vi "Example Interrupt.vi"() -> ()   [LabVIEW 2013]
uses:
  C:/tf/play/labview/Tinkerforge.dll
panel:
  out "value mask":bool[](array[boolean])
  out "interrupt mask":bool[](array[boolean])
  in  "stop":bool
  in  "uid":string="aE7"
  in  "port":i32=4223
  in  "host":string="localhost"
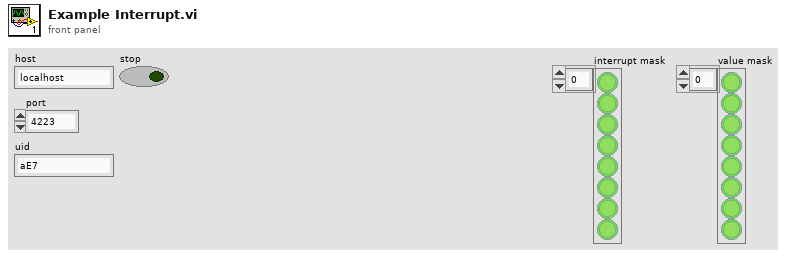
[diagram p1: front panel]
types:
  T1 = cluster{"port":u16, "interruptMask":u8, "valueMask":u8}
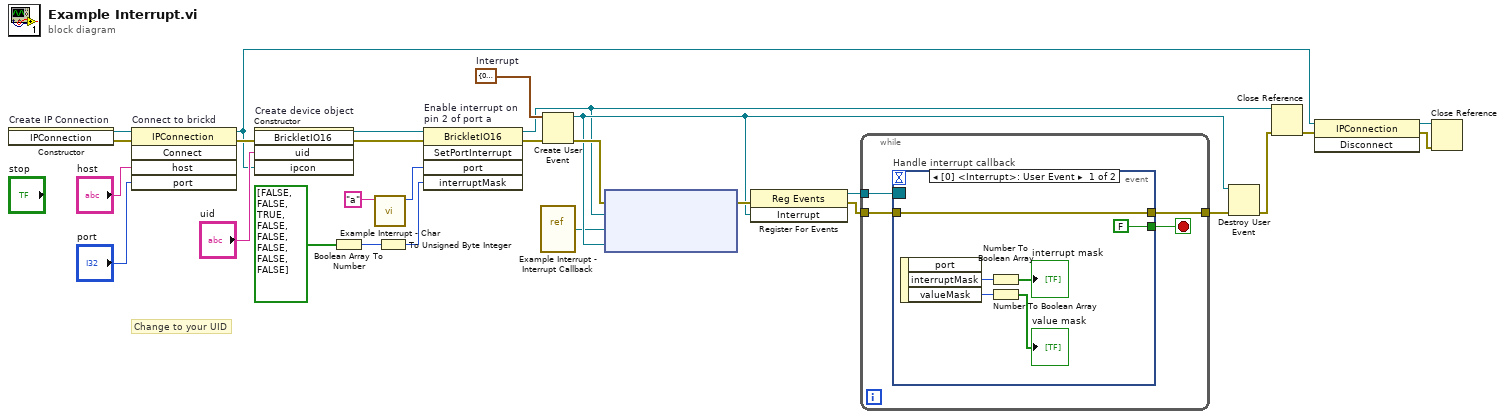
[diagram p0: block diagram]
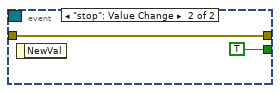
[diagram p2: hidden frame]
diagram:
  w12 = T1 {"port"=0, "interruptMask"=0, "valueMask"=0}  # Interrupt
  # "Change to your UID"
  n1 = constructor on="Create IP Connection" class="IPConnection"() -> (reference out=w28:refnum<k24>, error out=w7:errorcluster)  [unwired: 3 in, 1 out]
  n2 = invoke on="Connect to brickd" class="IPConnection" method="Connect"(reference=w28, error in=w7, "host"="host", "port"="port") -> (reference out=w21:refnum<k24>, error out=w24:errorcluster)  [unwired: 1 in, 3 out]
  n3 = constructor on="Create device object" class="BrickletIO16"(error in=w24, "uid"="uid", "ipcon"=w21) -> (reference out=w9:refnum<k24>, error out=w11:errorcluster)  [unwired: 2 in, 3 out]
  n4 = Boolean Array To Number(Boolean array=bool[] [FALSE, FALSE, TRUE, FALSE, FALSE, FALSE, FALSE, FALSE]) -> (number=w4:u32)
  n5 = call "Example Interrupt - Char.vi"("string"="a") -> ("char"=w2:u16)  [unwired: 10 in]
  n6 = To Unsigned Byte Integer(number=w4) -> (unsigned 8bit integer=w3:u8)
  n7 = invoke on="Enable interrupt on\npin 2 of port a" class="BrickletIO16" method="SetPortInterrupt"(reference=w9, error in=w11, "port"=w2, "interruptMask"=w3) -> (reference out=w8:refnum<k24>, error out=w10:errorcluster)  [unwired: 1 in, 3 out]
  n8 = vi-ref "Example Interrupt - Interrupt Callback.vi"() -> ("vi reference"=w1:refnum<vi>)
  n9 = Create User Event(user event datatype=w12, error in=w10) -> (user event=w14:refnum<user-event>, error out=w19:errorcluster)
  n10 = node ("Register Event Callback")(w19, w8, w1, w14) -> (w18:errorcluster)  [unwired: 1 in, 1 out]
  n11 = register-events(error in=w18, w14) -> (reference out=w17:refnum<event-registration>, error out=w15:errorcluster)  [unwired: 1 in]
  n12 = while {
    tunnel: w17 -> [w32]
    tunnel: [w31] -> w16
    tunnel: w15 -> [w30]
    stop <- w29 stop-if-true
    n13 = event "Handle interrupt callback" shown="[0] <Interrupt>: User Event" {
      selector: w32 -> [_ _]
      dyn-events: _ -> [_ _]
      timeout: _ -> [_ _]
      tunnel: [w38 w39] -> w31
      tunnel: w30 -> [w38 w39]
      tunnel: [FALSE TRUE] -> w29
      event User Event {
        n14 = event-data() -> ("interruptMask"=w33:u8, "valueMask"=w36:u8)  [unwired: 1 in, 1 out]
        n15 = Number To Boolean Array(number=w33) -> (Boolean array=→"interrupt mask":bool[])
        n16 = Number To Boolean Array(number=w36) -> (Boolean array=→"value mask":bool[])
      }
      event "stop": Value Change {
        n17 = event-data() -> ()  [unwired: 1 in, 1 out]
      }
    }
  }
  n18 = Destroy User Event(user event=w14, error in=w16) -> (error out=w13:errorcluster)
  n19 = Close Reference(reference=w8, error in (no error)=w13) -> (error out=w23:errorcluster)
  n20 = invoke class="IPConnection" method="Disconnect"(reference=w21, error in=w23) -> (reference out=w20:refnum<k24>, error out=w22:errorcluster)  [unwired: 1 in, 1 out]
  n21 = Close Reference(reference=w20, error in (no error)=w22) -> ()  [unwired: 1 out]
